vi "Match Channels to HW and Data.vi"(7 "Data Setup":refnum<vi>, 8 "error in (no error)":errorcluster, 11 "DAQmx Task Name":refnum<k21>) -> (0 "error IO":errorcluster, 2 "Data":string, 3 "Header":string)   [LabVIEW 2017]
uses:
  <resource>/objmgr/daqmx.rc
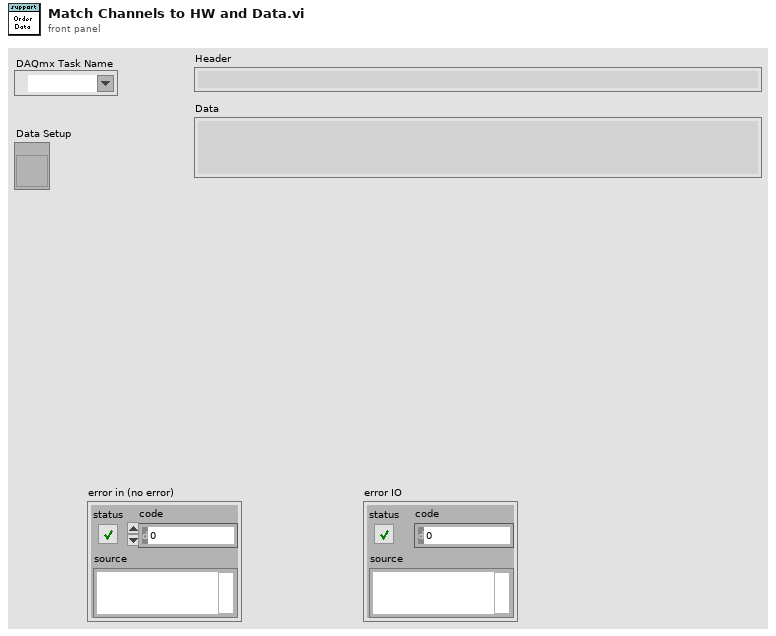
[diagram p1: front panel]
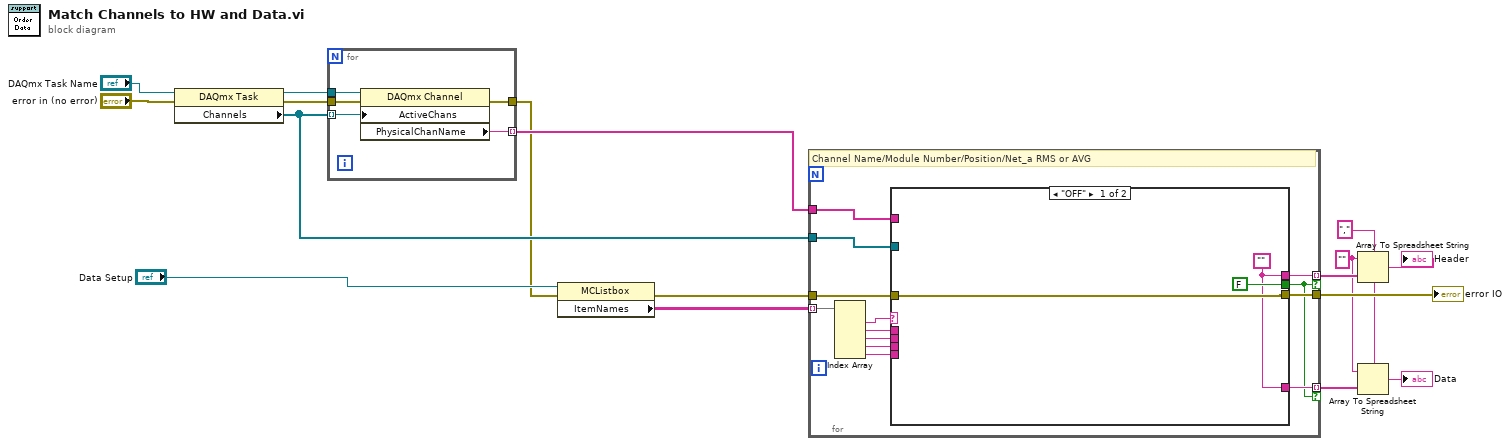
[diagram p0: block diagram]
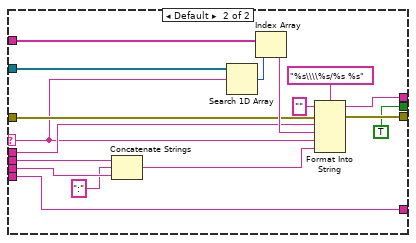
[diagram p2: hidden frame]
diagram:
  w1 = "" ("format string")
  w2 = "," ("delimiter (Tab)")
  n1 = property class="DAQmx Task"(reference="DAQmx Task Name", error in="error in (no error)") -> (reference out=w16:refnum<k21>, error out=w15:errorcluster, "Channels"=w12:refnum<k21>[])
  n2 = for {
    tunnel: w16 -> [w22]
    tunnel: w12 -> [w20] mode=indexing
    tunnel: w15 -> [w21]
    tunnel: [w19] -> w13 mode=indexing
    tunnel: [w18] -> w9
    n3 = property class="DAQmx Channel"(reference=w22, error in=w21, "ActiveChans"=w20) -> (error out=w18:errorcluster, "PhysicalChanName"=w19:tag)  [unwired: 1 out]
  }
  n4 = property on="Property Node" class="MCListbox"(reference="Data Setup", error in=w9) -> (error out=w8:errorcluster, "ItemNames"=w11:string[][])  [unwired: 1 out]
  n5 = for {
    tunnel: w11 -> [w35] mode=indexing
    tunnel: w12 -> [w34]
    tunnel: w13 -> [w33]
    tunnel: [w29] -> w5 mode=indexing if=w23
    tunnel: w8 -> [w28]
    tunnel: [w27] -> w7
    tunnel: [w31] -> w4 mode=indexing if=w23
    # "Channel Name/Module Number/Position/Net_a RMS or AVG"
    n6 = Index Array(array=w35) -> (element #1=w24:string, element #2=w32:string, element #3=w26:string, element #4=w25:string, element #5=w30:string)  [unwired: 5 in]
    n7 = case shown="\"OFF\"" w24 {
      selector: w24 -> [_ w45]
      tunnel: w34 -> [_ w55]
      tunnel: w33 -> [_ w54]
      tunnel: w32 -> [_ w51]
      tunnel: [w36 w39] -> w31
      tunnel: w30 -> [_ w39]
      tunnel: [w36 w49] -> w29
      tunnel: w28 -> [w38 w47]
      tunnel: [w38 w46] -> w27
      tunnel: w26 -> [_ w44]
      tunnel: w25 -> [_ w43]
      tunnel: [FALSE TRUE] -> w23
      frame "OFF" {
        w36 = ""
      }
      frame Default {
        n8 = Concatenate Strings(w44, ":", w43) -> (w42:string)
        n9 = Search 1D Array(1D array=w55, element=w45) -> (index of element=w50:i32)  [unwired: 1 in]
        n10 = Index Array(array=w54, index=w50) -> (element=w52:tag)
        n11 = Format Into String(format string="%s\\\\%s/%s %s", initial string="", error in=w47, w51, w52, w45, w42) -> (resulting string=w49:string, error out=w46:errorcluster)
      }
    }
  }
  "error IO" <- w7
  n12 = Array To Spreadsheet String(delimiter (Tab)=w2, array=w5, 3:w1) -> (spreadsheet string=→"Header":string)
  n13 = Array To Spreadsheet String(delimiter (Tab)=w2, array=w4, 3:w1) -> (spreadsheet string=→"Data":string)
